vi "Destroy.vi"(8 "error in (no error)":errorcluster, 11 "Deferer in":refnum<class "Deferer.lvclass">) -> (0 "error out":errorcluster)   [LabVIEW 2020, in "Panel.lvlib" / "Deferer.lvclass"]
doc: "Cleans up the deferer object. Panel updates will be undefered for the associated VI.\n\n----\nPlease see the following web address for additional documentation and tutorial information:\nhttp://www.mooregoodideas.com/mgi-panel-manager/\n\nAuthor: Derek Trepanier\n\nCopyright (c) 2018, Moore Good Ideas, Inc.\n\nAll rights reserved.\n\nRedistribution and use in source and binary forms, with or without modification, are permitted provided that the following conditions are met:\n\n * Redistributions of source code must retain the above copyright notice, this list of conditions and the following disclaimer.\n * Redistributions in binary form must reproduce the above copyright notice, this list of conditions and the following disclaimer in the documentation and/or other materials provided with the distribution.\n * Neither the name of Moore Good Ideas, Inc. nor the names of its contributors may be used to endorse or promote products derived from this software without specific prior written permission.\n\nTHIS SOFTWARE IS PROVIDED BY THE COPYRIGHT HOLDERS AND CONTRIBUTORS \"AS IS\" AND ANY EXPRESS OR IMPLIED WARRANTIES, INCLUDING, BUT NOT LIMITED TO, THE IMPLIED WARRANTIES OF MERCHANTABILITY AND FITNESS FOR A PARTICULAR PURPOSE ARE DISCLAIMED. IN NO EVENT SHALL THE COPYRIGHT OWNER OR CONTRIBUTORS BE LIABLE FOR ANY DIRECT, INDIRECT, INCIDENTAL, SPECIAL, EXEMPLARY, OR CONSEQUENTIAL DAMAGES (INCLUDING, BUT NOT LIMITED TO, PROCUREMENT OF SUBSTITUTE GOODS OR SERVICES; LOSS OF USE, DATA, OR PROFITS; OR BUSINESS INTERRUPTION) HOWEVER CAUSED AND ON ANY THEORY OF LIABILITY, WHETHER IN CONTRACT, STRICT LIABILITY, OR TORT (INCLUDING NEGLIGENCE OR OTHERWISE) ARISING IN ANY WAY OUT OF THE USE OF THIS SOFTWARE, EVEN IF ADVISED OF THE POSSIBILITY OF SUCH DAMAGE."
uses:
  <vilib>/MGI/Panel Manager/Panel/Deferer/Deferer.lvclass
  <vilib>/MGI/Panel Manager/Panel/Deferer/Deferer.lvclass/Deferer.ctl
  <vilib>/MGI/Panel Manager/Panel/Panel Control Counter/Panel Control Counter.lvclass
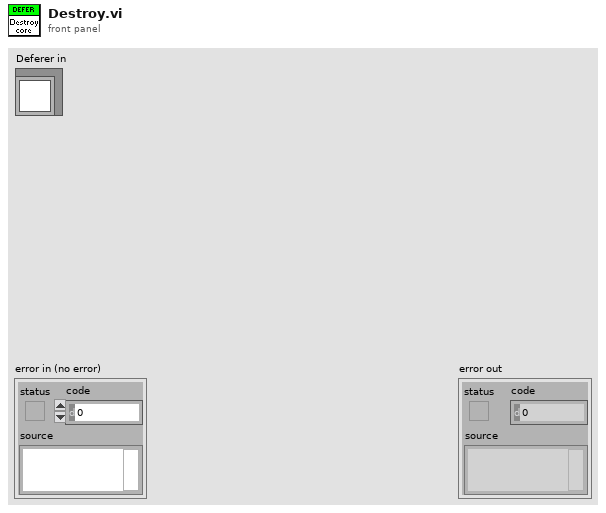
[diagram p1: front panel]
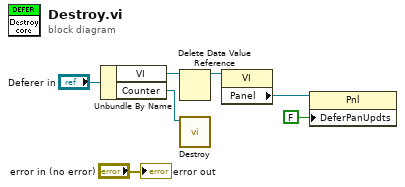
[diagram p0: block diagram]
diagram:
  n1 = Unbundle By Name("Deferer in") -> ("VI"=w5:refnum<data-value>, "Counter"=w1:refnum<class "Panel Control Counter.lvclass">)
  n2 = Delete Data Value Reference(data value reference=w5) -> (data value=w3:refnum<vi>)  [unwired: 1 in, 1 out]
  n3 = call <vilib>:"Destroy.vi"("Panel Control Counter in"=w1) -> ()  [unwired: 10 in, 1 out]
  n4 = property class="VI"(reference=w3) -> ("Panel"=w4:refnum<vi>)  [unwired: 1 in, 2 out]
  n5 = property class="Pnl"(reference=w4, "DeferPanUpdts"=FALSE ("Defer Panel Updates")) -> ()  [unwired: 1 in, 2 out]
  "error out" <- "error in (no error)"
